vi "Real time state machine - Saccade suppression LED by time2.vi"() -> ()   [LabVIEW 2013]
uses:
  <vilib>/Platform/TimedLoop/XDataNode/timing_clust.ctl
  <vilib>/Platform/TimedLoop/XDataNode/nitl_modes.ctl
  <vilib>/Platform/TimedLoop/XDataNode/wakeup.ctl
  <vilib>/DAQmx/write.llb/DAQmx Write (Digital 1D Bool NChan 1Samp 1Line).vi
  <vilib>/DAQmx/read.llb/DAQmx Read (Analog 1D DBL NChan 1Samp).vi
  <vilib>/DAQmx/write.llb/DAQmx Write (Analog DBL 1Chan 1Samp).vi
  <vilib>/platform/TimedLoop/XDataNode/XDataNode.xnode
  <vilib>/Platform/TimedLoop/XDataNode/XDNodeRunTimeDep.lvlib
panel:
  in  "Local port":u16=9091
  in  "Local IP_This computer":string="192.168.137.2"
  out "ABORT":bool
  out "Initial data received":bool
  out "Busy":bool
  out "Trial Done":bool=TRUE
  in  "Remote port":u16=9090
  in  "Remote IP_Main":string="192.168.137.10"
  out "Trial #":i32=5
  out "Start one trial":bool
  out "RT FIFO (Log)":u32(slide) scale=0.0..50.0
  out "error out":errorcluster
  out "Actual cycle period (uS)":i64=104
  out "# of rewards":i32
  in  "Automatic reward":bool=TRUE
  out "Digital Waveform Graph":digitalwaveform(graph)={"t0"=timestamp(3672173571.3850894 s since 1904-01-01), "dt"=0.0004, "Y"={"transitions"=[], "data"=array25000x3[75000 elements]}, "error"={"status"=FALSE, "code"=37421928, "source"=""}}
  out "shaft encoder":waveform(sgl)(graph)={"t0"=timestamp(3672173571.3850894 s since 1904-01-01), "dt"=0.02, "Y"=array[500 elements]}
  out "Min":dbl=20.0
  out "Sec":dbl=23.69873046875
  out "Trial # (State machine)":u32=6
  out "Current state":T1(ring)
  out "RT FIFO (DISP)":u32(slide) scale=0.0..50.0
  in  "State machine cycle (uS)":i64=200
  in  "Save file to":string="C:\\ni-rt\\LabVIEW Data\\"
  in  "Display length (S)":sgl=10.0
  in  "RT FIFO size":u32=50
  in  "VS filter period (uS)":i32=500
  out "LED?":bool
  out "Pulse amp 0":sgl
  out "Pulse amp 1":sgl
  out "Pulse delay":sgl
  out "Pulse width":sgl
  out "Pulse period (ms)":sgl
  out "Pulse #":sgl
  out "Reward period (uS)":u32
  out "Reward start delay (uS)":u32
  out "Water duration (uS)":u32=30000
  out "Water refractory period (uS)":u32=500000
  out "Shock duration (uS)":u32=10000
  out "Shock refractory period (uS)":u32=1000000
  out "Trial timeout (uS)":u32=3000000
  out "Lick threshold (V)":fxp<+,32,16>=1.600006103515625
  out "Track eye":bool=TRUE
  out "Allow shock":bool
  out "Allow timeout":bool
  out "Manually give water":bool
  out "Manually give shock":bool
  out "VS threshold (V)":fxp<+,32,16>=2.0
  out "VS type":string="test"
  out "File name":string="Test"
  out "Behavior type":string="test"
  out "Save data":bool
  out "Lick reward":bool
  in  "Stop state":bool
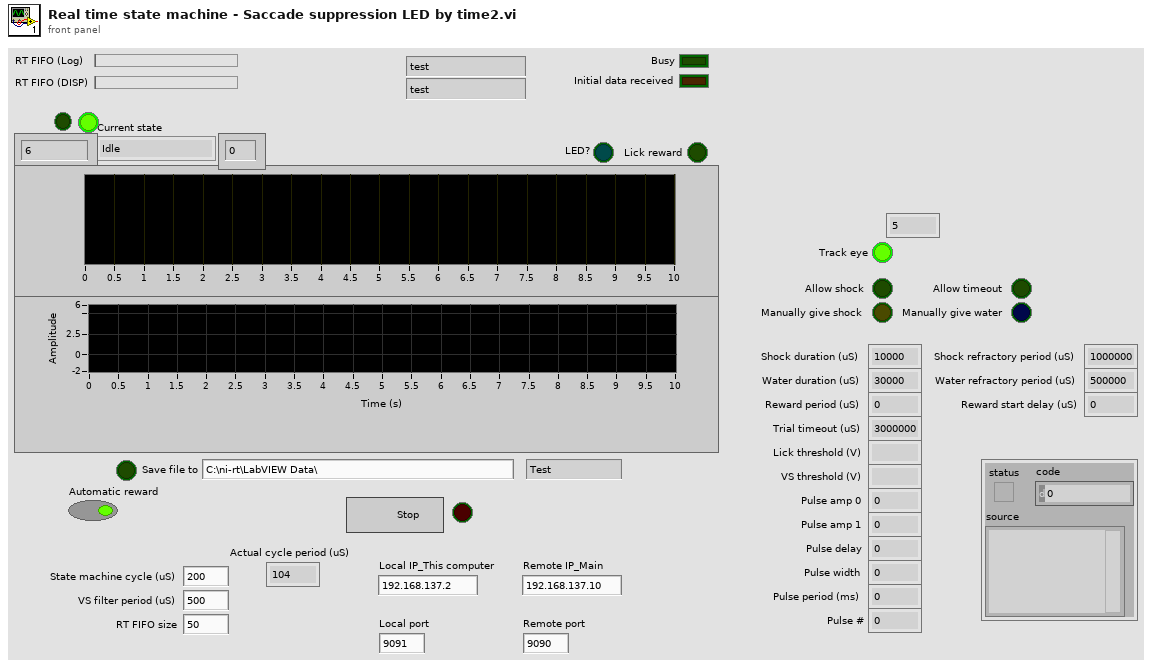
[diagram p1: front panel]
types:
  T1 = enum16{"Idle", "Before VS", "VS", "VS2", "After VS", "Wait for lever press", "Cycle End", "Reward", "Reward Refractory", "Punish", "Punish Refractory", "Exit", "Timeout", "Lick reward"}
  T2 = enum16{"open", "replace", "create", "open or create", "replace or create", "replace or create with confirmation"}
  T3 = typedef "XDNodeRunTimeDep.lvlib/timing_clust.ctl" = cluster{"Expected End [f-1]":u64, "Actual End [f-1]":u64, "Finished Late? [f-1]":bool, "Expected End [i-1]":u64, "Actual End [i-1]":u64, "Finished Late? [i-1]":bool, "Expected Start [i]":u64, "Actual Start [i]":u64, "Expected Start [f]":u64, "Actual Start [f]":u64, "Source Name":string, "Structure Name":string, "Period":i64, "Deadline":i64, "Offset":i64, "Start":i64, "Priority":i32, "Timeout":i32, "Mode":T4, "Wakeup Reason":T5, "Error":errorcluster, "Source Type":string, "Secondary Source Type":string, "Global End Time":u64, "Global Start Time":u64, "Frame Duration":u64, "Iteration Duration":u64, "Assigned CPU":i32, "I/O Scan Engine Mode":u32}
  T4 = typedef "XDNodeRunTimeDep.lvlib/nitl_modes.ctl" = enum32{"No Change", "Process missed periods, maintain original phase", "Discard missed periods, maintain original phase", "Process missed periods, ignore original phase", "Discard missed periods, ignore original phase"}
  T5 = typedef "XDNodeRunTimeDep.lvlib/wakeup.ctl" = enum32{"Normal", "Aborted", "Asynchronous wakeup", "Timing source error", "Timed loop error", "Timeout"}
  T6 = enum16{"big-endian, network order", "native, host order", "little-endian"}
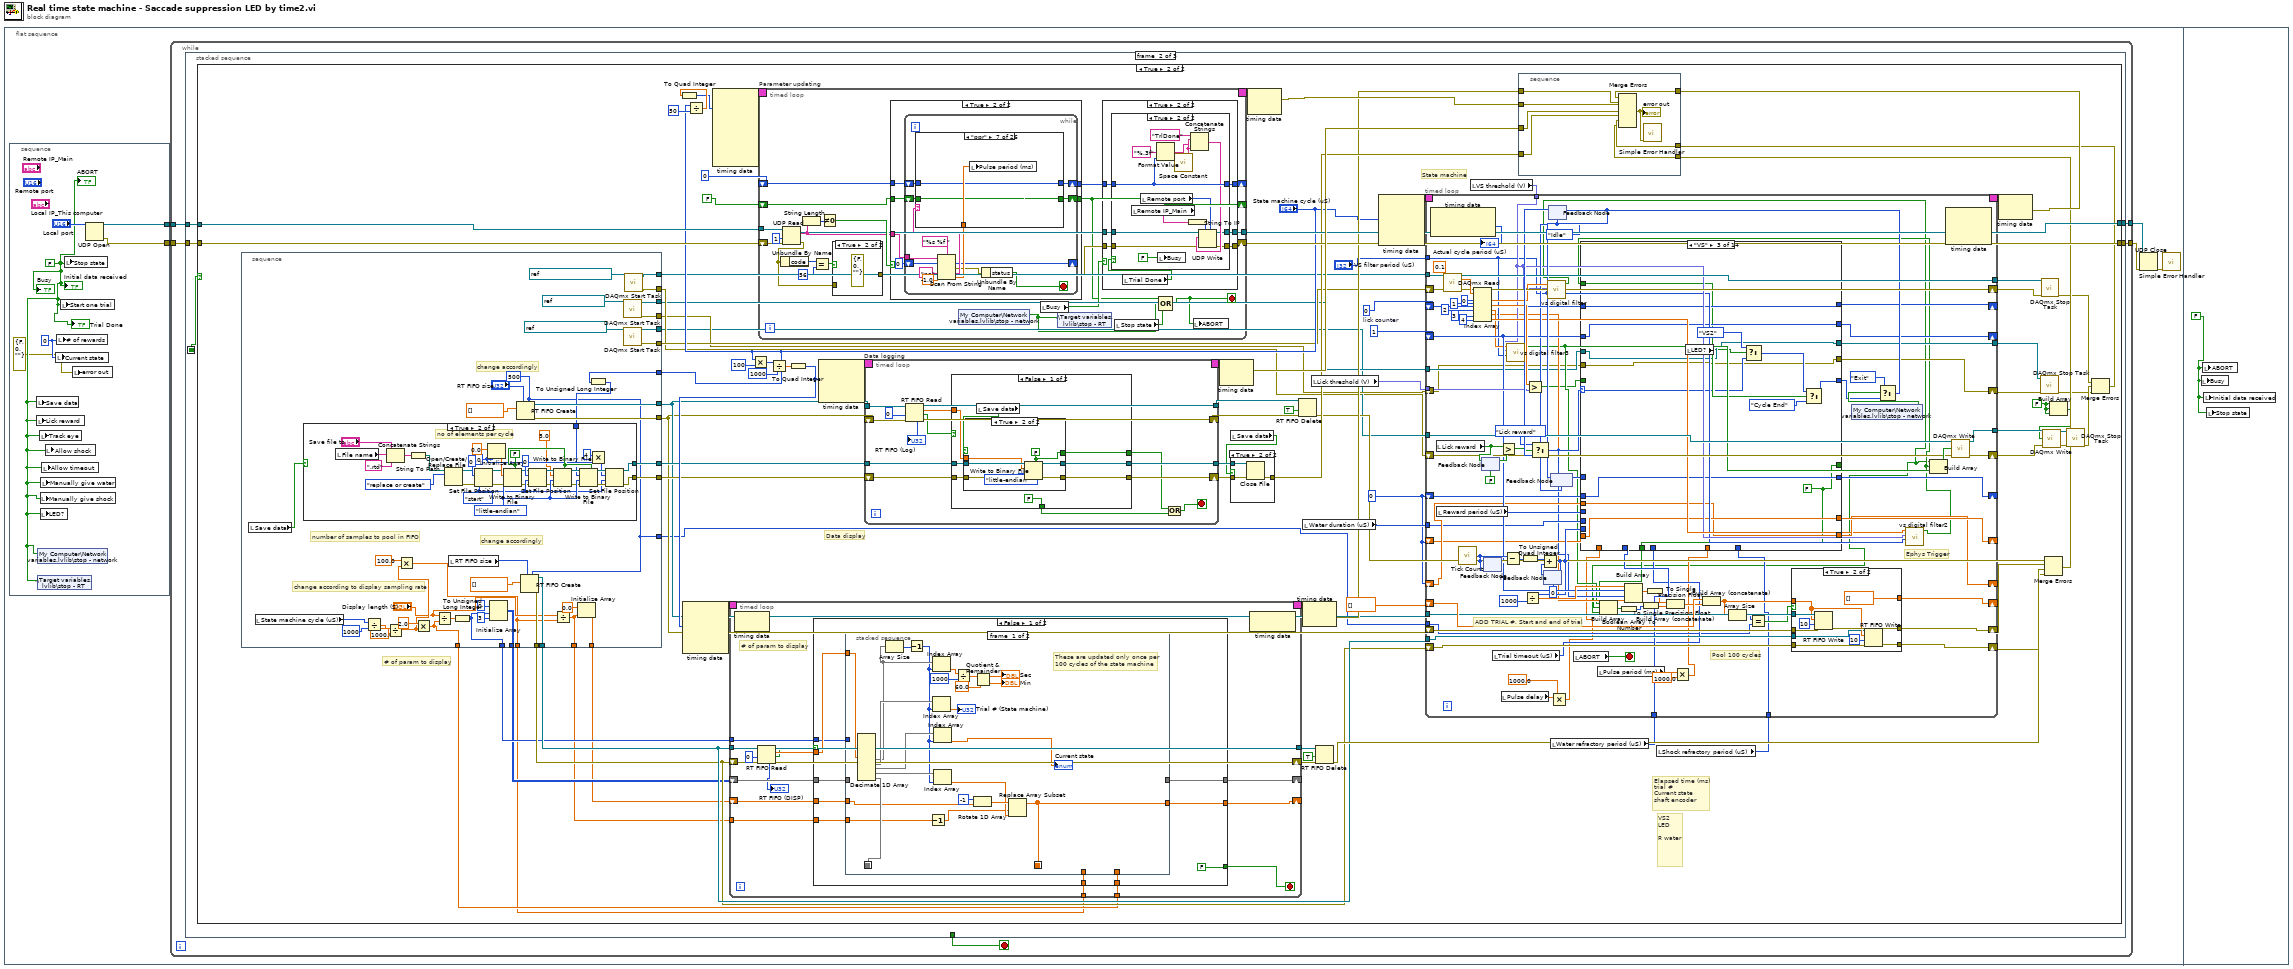
[diagram p0: block diagram]
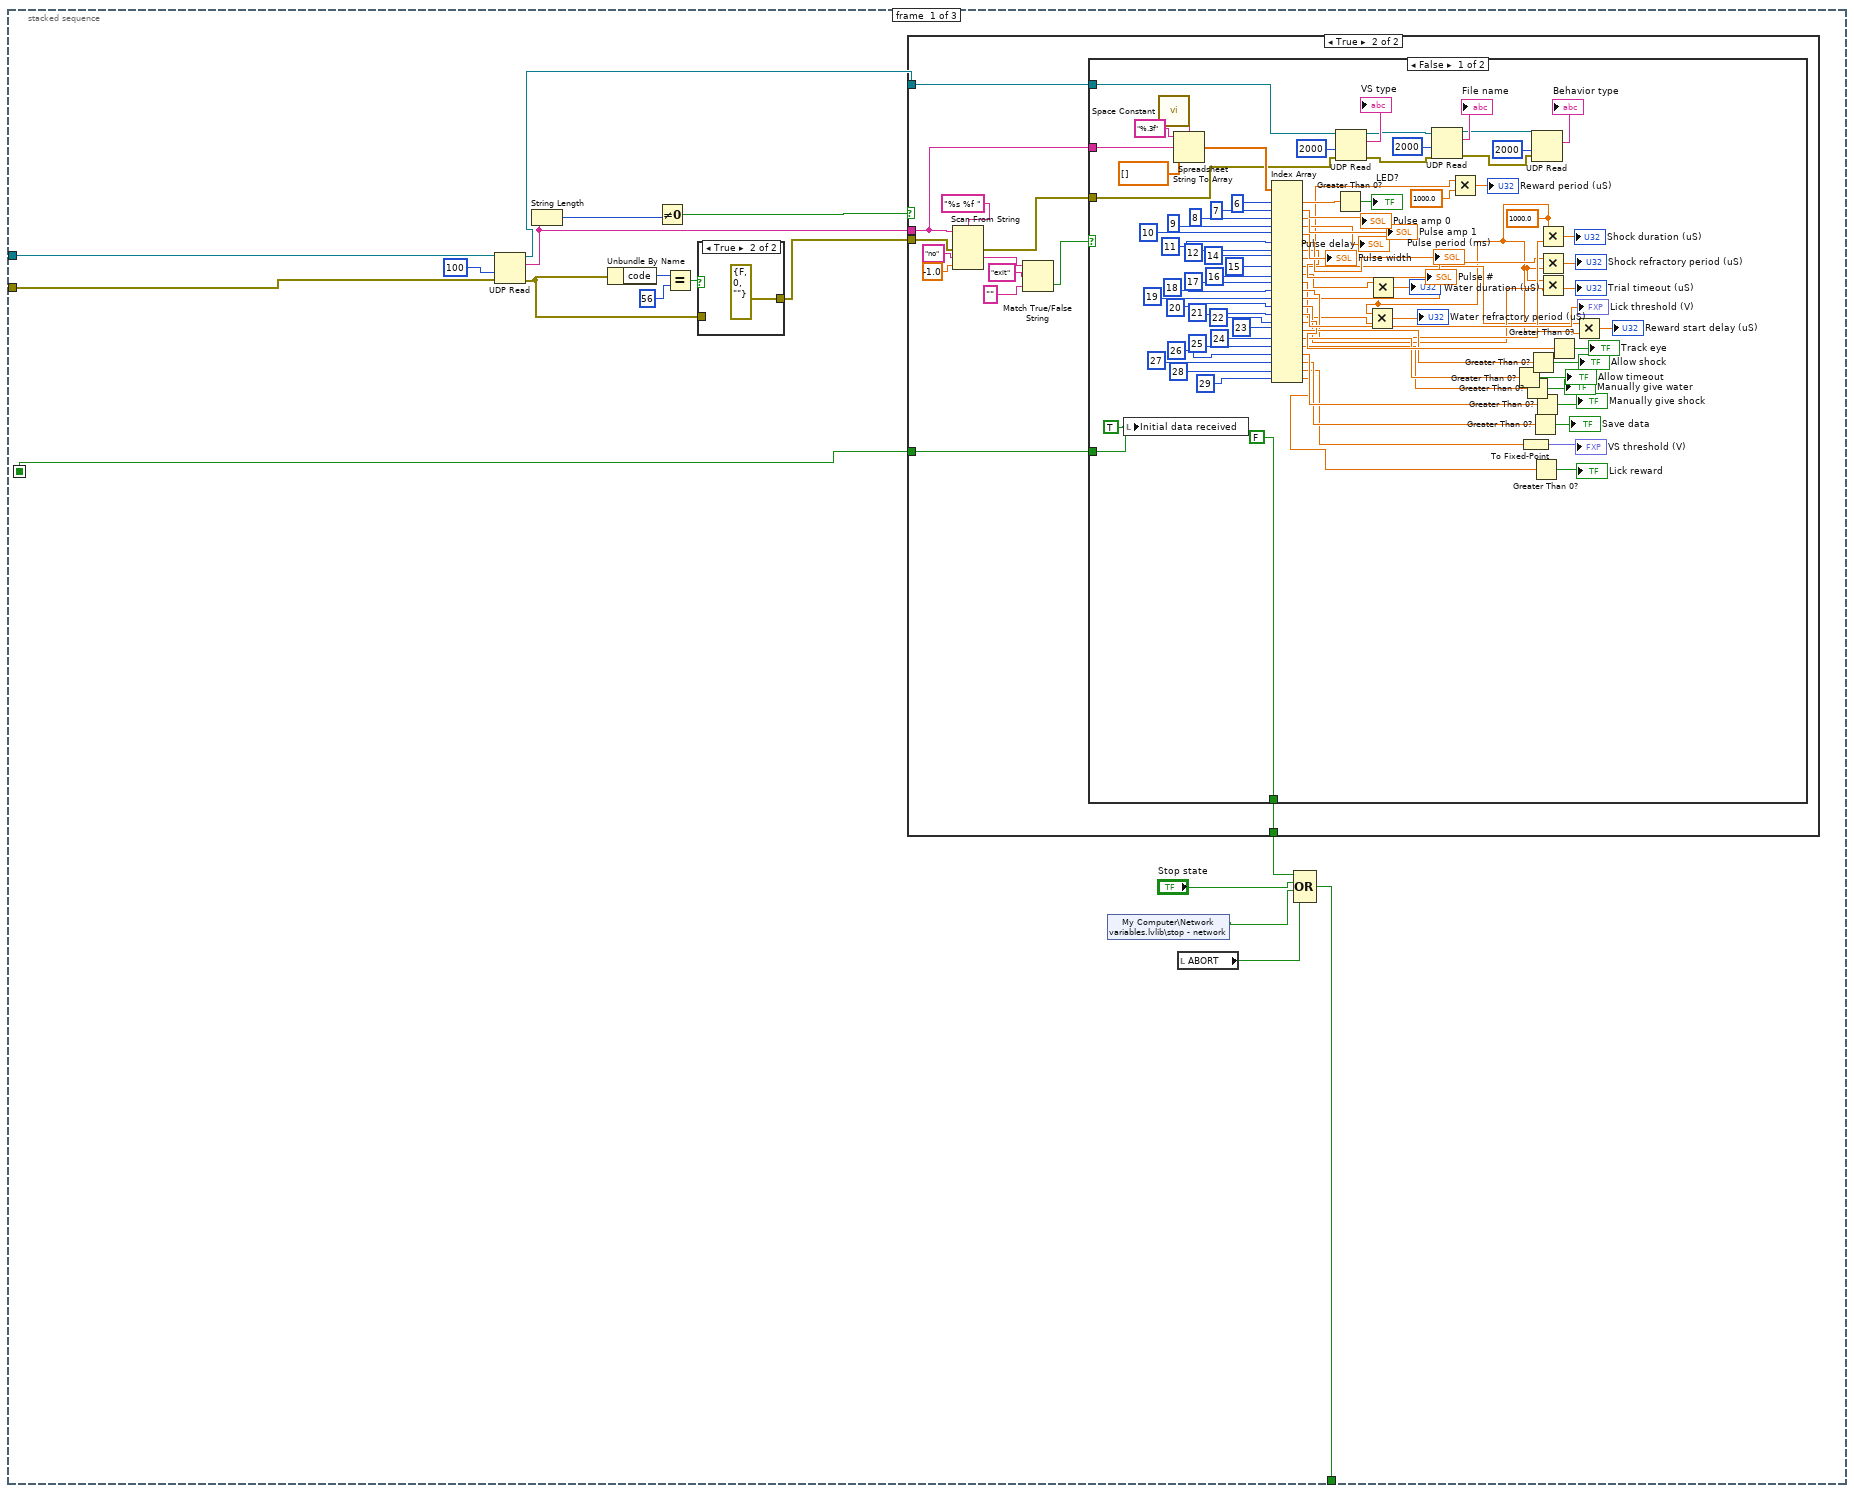
[diagram p2: hidden frame]
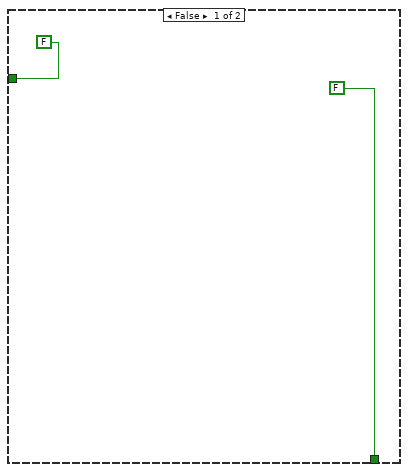
[diagram p3: hidden frame]
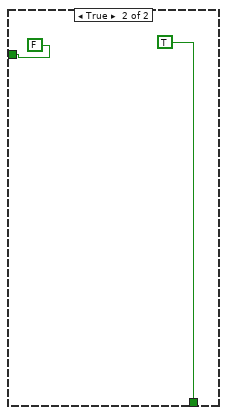
[diagram p4: hidden frame]
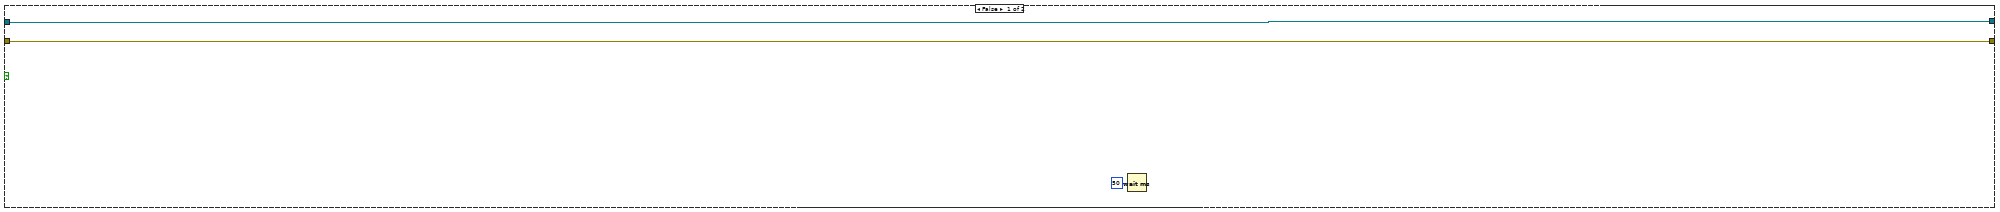
[diagram p6: hidden frame]
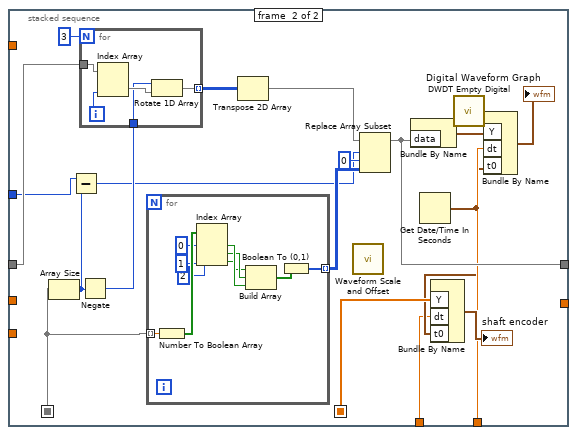
[diagram p9: hidden frame]
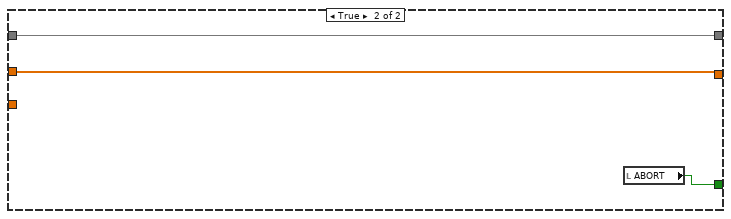
[diagram p10: hidden frame]
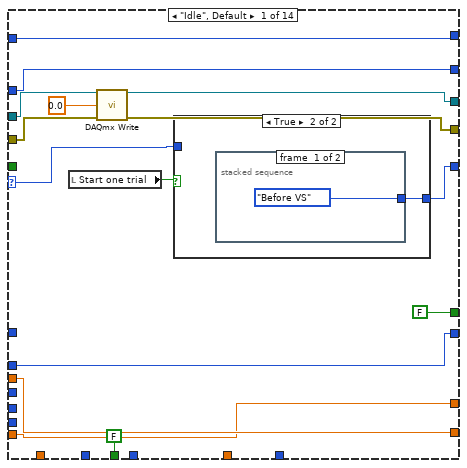
[diagram p11: hidden frame]
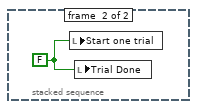
[diagram p13: hidden frame]
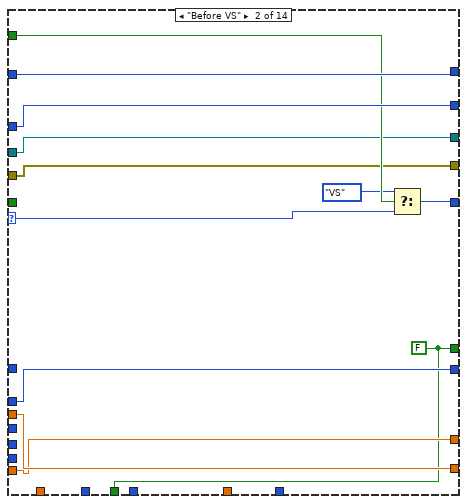
[diagram p14: hidden frame]
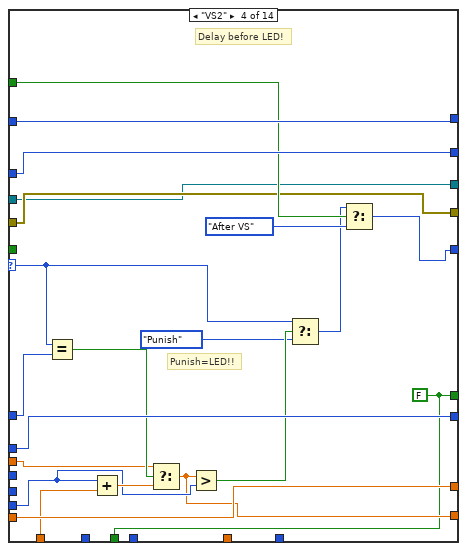
[diagram p15: hidden frame]
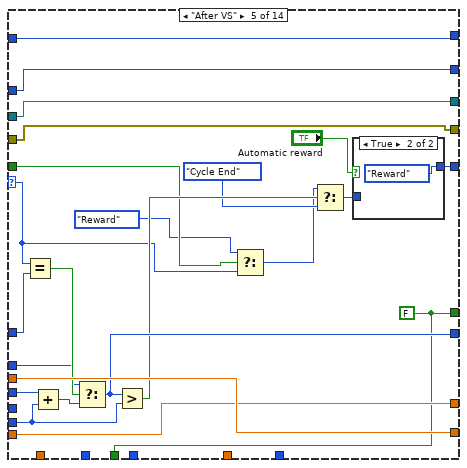
[diagram p16: hidden frame]
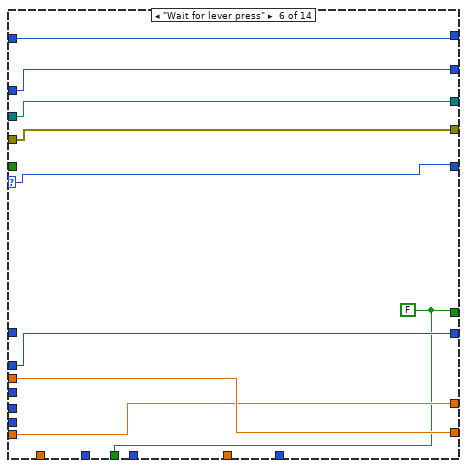
[diagram p18: hidden frame]
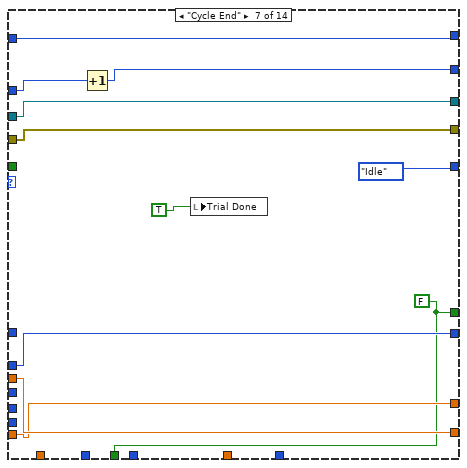
[diagram p19: hidden frame]
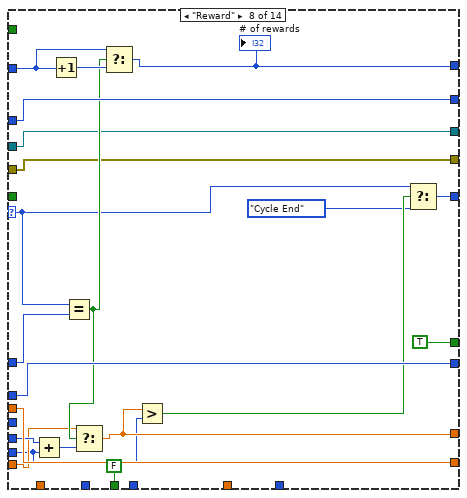
[diagram p20: hidden frame]
diagram:
  n1 = flat-sequence {
    frame #0 {
      n2 = stacked-sequence {
        tunnel: [w995] -> w5
        tunnel: [w994] -> w4
        frame #0 {
          w993 = 0
          w992 = FALSE
          n3 = local write "Save data"(w992) -> ()
          n4 = local write "Lick reward"(w992) -> ()
          n5 = shared-variable "My Computer\\Network variables.lvlib\\stop - network"(w992) -> ()  [unwired: 1 in, 1 out]
          n6 = shared-variable ".\\Target variables.lvlib\\stop - RT"(w992) -> ()  [unwired: 1 in, 1 out]
          n7 = local write "Track eye"(w992) -> ()
          n8 = local write "Manually give shock"(w992) -> ()
          n9 = local write "LED?"(w992) -> ()
          n10 = local write "Manually give water"(w992) -> ()
          n11 = local write "Allow timeout"(w992) -> ()
          n12 = local write "Allow shock"(w992) -> ()
          n13 = local write "Current state"(w993) -> ()
          n14 = local write "# of rewards"(w993) -> ()
          n15 = local write "Start one trial"(w992) -> ()
          n16 = local write "Stop state"(w992) -> ()
          n17 = local write "error out"(errorcluster {"status"=FALSE, "code"=0, "source"=""} ("error out")) -> ()
          n18 = UDP Open(11:"Local port") -> (port=w995:refnum<k16>, 0:w994:errorcluster)  [unwired: 4 in, 1 out]
          "ABORT" <- w992
          "Initial data received" <- w992
          "Busy" <- w992
          "Trial Done" <- w992
        }
      }
      n19 = while {
        tunnel: w5 -> [w10]
        tunnel: w4 -> [w9]
        tunnel: [w8] -> w3
        tunnel: [w7] -> w2
        stop <- w6 stop-if-true
        n20 = stacked-sequence {
          seq-local: [w16 _ _] -> [_ w135 _]
          tunnel: w10 -> [w27 w132 _]
          tunnel: w9 -> [w26 w133 _]
          tunnel: [w15 _ _] -> w6
          tunnel: [_ w134 _] -> w8
          tunnel: [_ w131 _] -> w7
          frame #0 {
            n21 = UDP Read(connection ID=w27, timeout ms (25000)=100, 8:w26) -> (data out=w18:string, error out=w22:errorcluster, 3:w17:refnum<k16>)  [unwired: 1 in, 2 out]
            n22 = String Length(string=w18) -> (length=w21:i32)
            n23 = Unbundle By Name(w22) -> ("code"=w25:i32)
            n24 = Not Equal To 0?(x=w21) -> (x != 0?=w20:bool)
            n25 = Equal?(x=w25, y=56) -> (x = y?=w23:bool)
            n26 = case shown="True" w23 {
              tunnel: w22 -> [w129 _]
              tunnel: [w129 errorcluster {"status"=FALSE, "code"=0, "source"=""} ("error out")] -> w19
              frame False {
              }
              frame True {
              }
            }
            n27 = case shown="True" w20 {
              tunnel: w19 -> [_ w41]
              tunnel: w18 -> [_ w35]
              tunnel: w17 -> [_ w33]
              tunnel: [FALSE w32] -> w14
              tunnel: [FALSE w31] -> w16
              frame False {
              }
              frame True {
                n28 = Scan From String(format string="%s %f ", input string=w35, error in=w41, default 1="no" ("default value 1"), default 2=sgl -1.0 ("default value 1")) -> (error out=w34:errorcluster, output 1=w39:string)  [unwired: 2 in, 2 out]
                n29 = Match True/False String(2:"" ("false string"), 3:"exit" ("true string"), 4:w39) -> (0:w36:bool)  [unwired: 1 out]
                n30 = case shown="False" w36 {
                  tunnel: w35 -> [w123 _]
                  tunnel: w34 -> [w81 _]
                  tunnel: w33 -> [w80 _]
                  tunnel: [FALSE TRUE] -> w32
                  tunnel: [w68 FALSE] -> w31
                  frame False {
                    w49 = sgl 1000.0
                    w68 = TRUE
                    n31 = local write "Initial data received"(w68) -> ()
                    n32 = call <vilib>:"Space Constant.vi"() -> ("String"=w125:string)
                    n33 = Spreadsheet String To Array(delimiter (Tab)=w125, format string="%.3f", spreadsheet string=w123, array type (2D Dbl)=sgl[] []) -> (array=w122:sgl[])
                    n34 = Index Array(array=w122, index #1=6 ("index"), index #2=7 ("index"), index #3=8 ("index"), index #4=9 ("index"), index #5=10 ("index"), index #6=11 ("index"), index #7=12 ("index"), index #8=14 ("index"), index #9=15 ("index"), index #10=16 ("index"), index #11=17 ("index"), index #12=18 ("index"), index #13=19 ("index"), index #14=20 ("index"), index #15=21 ("index"), index #16=22 ("index"), index #17=23 ("index"), index #18=24 ("index"), index #19=25 ("index"), index #20=26 ("index"), index #21=27 ("index"), index #22=28 ("index"), index #23=29 ("index")) -> (element #1=w120:sgl, element #2=→"Pulse amp 0":sgl, element #3=→"Pulse amp 1":sgl, element #4=→"Pulse delay":sgl, element #5=→"Pulse width":sgl, element #6=→"Pulse period (ms)":sgl, element #7=→"Pulse #":sgl, element #8=w64:sgl, element #9=w55:sgl, element #10=w53:sgl, element #11=w51:sgl, element #12=w61:sgl, element #13=w60:sgl, element #14=w57:sgl, element #15=→"Lick threshold (V)":sgl, element #16=w94:sgl, element #17=w91:sgl, element #18=w89:sgl, element #19=w86:sgl, element #20=w84:sgl, element #21=w46:sgl, element #22=w45:sgl, element #23=w44:sgl)
                    n35 = Greater Than 0?(x=w120) -> (x > 0?=→"LED?":bool)
                    n36 = UDP Read(connection ID=w80, timeout ms (25000)=2000, 8:w81) -> (data out=→"VS type":string, error out=w76:errorcluster, 3:w74:refnum<k16>)  [unwired: 1 in, 2 out]
                    n37 = Multiply(x=w49, y=w51) -> (x*y=→"Water refractory period (uS)":sgl)
                    n38 = Multiply(x=w53, y=w49) -> (x*y=→"Water duration (uS)":sgl)
                    n39 = UDP Read(connection ID=w74, timeout ms (25000)=2000, 8:w76) -> (data out=→"File name":string, error out=w72:errorcluster, 3:w71:refnum<k16>)  [unwired: 1 in, 2 out]
                    n40 = Multiply(x=w64, y=sgl 1000.0) -> (x*y=→"Reward period (uS)":sgl)
                    n41 = Greater Than 0?(x=w89) -> (x > 0?=→"Allow timeout":bool)
                    n42 = To Fixed-Point(number=w45) -> (fixed-point=→"VS threshold (V)":fxp<+/-,32,16>)  [unwired: 1 in]
                    n43 = Greater Than 0?(x=w86) -> (x > 0?=→"Manually give water":bool)
                    n44 = Greater Than 0?(x=w91) -> (x > 0?=→"Allow shock":bool)
                    n45 = Greater Than 0?(x=w46) -> (x > 0?=→"Save data":bool)
                    n46 = Greater Than 0?(x=w44) -> (x > 0?=→"Lick reward":bool)
                    n47 = UDP Read(connection ID=w71, timeout ms (25000)=2000, 8:w72) -> (data out=→"Behavior type":string)  [unwired: 1 in, 4 out]
                    n48 = Greater Than 0?(x=w84) -> (x > 0?=→"Manually give shock":bool)
                    n49 = Multiply(x=w49, y=w61) -> (x*y=→"Shock duration (uS)":sgl)
                    n50 = Multiply(x=w60, y=w49) -> (x*y=→"Shock refractory period (uS)":sgl)
                    n51 = Multiply(x=w49, y=w57) -> (x*y=→"Trial timeout (uS)":sgl)
                    n52 = Greater Than 0?(x=w94) -> (x > 0?=→"Track eye":bool)
                    n53 = Multiply(x=w55, y=w49) -> (x*y=→"Reward start delay (uS)":sgl)
                  }
                  frame True {
                  }
                }
              }
            }
            n54 = shared-variable "My Computer\\Network variables.lvlib\\stop - network"() -> (w11:bool)  [unwired: 1 in, 1 out]
            n55 = local read "ABORT"() -> (w12:bool)
            n56 = Compound Arithmetic op=OR(w14, "Stop state", w11, w12) -> (w15:bool)
          }
          frame #1 {
            n57 = case shown="True" w135 {
              tunnel: w133 -> [w138 w215]
              tunnel: [w138 w207] -> w134
              tunnel: w132 -> [w137 w214]
              tunnel: [w137 w206] -> w131
              frame False {
                n58 = Wait (ms)(milliseconds to wait=u32 50) -> ()  [unwired: 1 out]
              }
              frame True {
                w159 = FALSE
                w195 = 0  # lick counter
                w152 = 0
                # "VS2\nLED\n\nR water"
                # "# of param to display"
                # "Data display"
                # "Elapsed time (ms)\ntrial #\nCurrent state\nshaft encoder"
                # "State machine"
                n59 = stacked-sequence {
                  tunnel: [w267] -> w180
                  tunnel: [w266] -> w179
                  tunnel: [w263] -> w178
                  tunnel: [w262] -> w177
                  tunnel: [w248] -> w160
                  tunnel: [w243] -> w176
                  tunnel: [w254] -> w175
                  tunnel: "State machine cycle (uS)" -> [w247]
                  tunnel: [w251] -> w173
                  tunnel: [w250] -> w172
                  tunnel: [w245] -> w151
                  tunnel: [w242] -> w150
                  tunnel: [w238] -> w149
                  tunnel: [w237] -> w148
                  tunnel: [w235] -> w144
                  tunnel: [w234] -> w143
                  tunnel: [w232] -> w142
                  tunnel: [w231] -> w141
                  tunnel: [w229] -> w140
                  tunnel: [w228] -> w139
                  frame #0 {
                    w245 = u32 500 ("elements in array (1)")
                    # "number of samples to pool in FIFO"
                    # "change according to display sampling rate"
                    # "change accordingly"
                    # "change accordingly"
                    n60 = local read "Save data"() -> (w268:bool)
                    n61 = local read "State machine cycle (uS)"() -> (w255:i64)
                    n62 = Divide(x=w255, y=u32 1000) -> (x/y=w257:dbl)
                    n63 = Divide(x=w257, y=1000.0) -> (x/y=w240:dbl)
                    n64 = Multiply(x=100.0, y=w240) -> (x*y=w238:dbl)
                    n65 = Multiply(x=2.0, y=w240) -> (x*y=w248:dbl)
                    n66 = Divide(x="Display length (S)", y=w248) -> (x/y=w260:dbl)
                    n67 = local read "RT FIFO size"() -> (w265:u32)
                    n68 = To Unsigned Long Integer(number=w260) -> (unsigned 32bit integer=w243:u32)
                    n69 = Initialize Array(u8 0 ("element"), w243, 3 ("dimension size")) -> (w254:u8[][])
                    n70 = RT FIFO Create(1:sgl[] [], 4:"RT FIFO size", 6:w245) -> (8:w251:refnum<k33>, 11:w250:errorcluster)  [unwired: 5 in, 1 out]
                    n71 = RT FIFO Create(1:sgl[] [], 4:w265, 6:w245) -> (8:w263:refnum<k33>, 11:w262:errorcluster)  [unwired: 5 in, 1 out]
                    n72 = Divide(x="Display length (S)", y=w238) -> (x/y=w237:dbl)
                    n73 = Initialize Array(sgl 0.0 ("element"), w237) -> (w242:sgl[])
                    n74 = To Unsigned Long Integer(number=w247) -> (unsigned 32bit integer=w246:u32)
                    n75 = case shown="True" w268 {
                      tunnel: [_ w272] -> w267
                      tunnel: [_ w271] -> w266
                      tunnel: w246 -> [_ w270]
                      frame False {
                      }
                      frame True {
                        w293 = FALSE
                        w286 = 10 ("dimension size")
                        w294 = T6."little-endian" ("byte order (0:big-endian, network order)")
                        w285 = enum16{"start", "end", "current"}."start" ("from (0:start)")
                        # "no of elements per cycle"
                        n76 = local read "File name"() -> (w296:string)
                        n77 = Concatenate Strings("Save file to", w296, ".rtd" ("string")) -> (w299:string)
                        n78 = String To Path(string=w299) -> (path=w300:path)
                        n79 = Open/Create/Replace File(file path (use dialog)=w300, operation (0:open)=T2."replace or create") -> (refnum out=w273:refnum<file>, error out=w274:errorcluster)  [unwired: 4 in, 1 out]
                        n80 = Set File Position(offset (in bytes) (0)=i64 0, refnum=w273, from (0:start)=w285, error in=w274) -> (refnum out=w276:refnum<file>, error out=w277:errorcluster)
                        n81 = Initialize Array(sgl 0.0 ("element"), w286) -> (w279:sgl[])
                        n82 = Write to Binary File(file (use dialog)=w276, data=w279, error in=w277, 5:w293, 9:w294) -> (refnum out=w281:refnum<file>, error out=w280:errorcluster)  [unwired: 1 in, 1 out]
                        n83 = Set File Position(offset (in bytes) (0)=i64 0, refnum=w281, from (0:start)=w285, error in=w280) -> (refnum out=w283:refnum<file>, error out=w284:errorcluster)
                        n84 = Write to Binary File(file (use dialog)=w283, data=sgl 5.0, error in=w284, 5:w293, 9:w294) -> (refnum out=w291:refnum<file>, error out=w289:errorcluster)  [unwired: 1 in, 1 out]
                        n85 = Write to Binary File(file (use dialog)=w291, data=w270, error in=w289, 5:w293, 9:w294) -> (refnum out=w292:refnum<file>, error out=w290:errorcluster)  [unwired: 1 in, 1 out]
                        n86 = Multiply(x=4, y=w286) -> (x*y=w288:i32)
                        n87 = Set File Position(offset (in bytes) (0)=w288, refnum=w292, from (0:start)=w285, error in=w290) -> (refnum out=w271:refnum<file>, error out=w272:errorcluster)
                      }
                    }
                    n88 = call <vilib>:"DAQmx Start Task.vi"("task/channels in"=refnum<k21> "LED analog out" ("DAQmx Task Name")) -> ("task out"=w232:refnum<k21>, "error out"=w231:errorcluster)  [unwired: 13 in]
                    n89 = call <vilib>:"DAQmx Start Task.vi"("task/channels in"=refnum<k21> "Digital_write_saccade" ("DAQmx Task Name")) -> ("task out"=w229:refnum<k21>, "error out"=w228:errorcluster)  [unwired: 13 in]
                    n90 = call <vilib>:"DAQmx Start Task.vi"("task/channels in"=refnum<k21> "Analog_read_saccade" ("DAQmx Task Name")) -> ("task out"=w235:refnum<k21>, "error out"=w234:errorcluster)  [unwired: 13 in]
                  }
                }
                n91 = Divide(x="State machine cycle (uS)", y=i64 50) -> (x/y=w185:dbl)
                n92 = To Quad Integer(1:w185) -> (0:w184:i64)
                n93 = node-c288 ("Input Node")(w184) -> (w223:T3)  [unwired: 6 in]
                n94 = Multiply(x="State machine cycle (uS)", y=u32 100) -> (x*y=w188:i64)
                n95 = timed-loop "Parameter updating" {
                  timing: w223 -> [_]
                  timing-out: [_] -> w222
                  tunnel: w214 -> [w828]
                  shift-right: [w813] -> w207
                  shift-left: w215 -> [w829]
                  shift-right: [w816] -> _
                  shift-left: 0 -> [w819]
                  tunnel: [w812] -> w206
                  shift-right: [w810] -> _
                  shift-left: FALSE -> [w820]
                  stop <- w811 stop-if-true
                  n96 = UDP Read(connection ID=w828, timeout ms (25000)=1, 8:w829) -> (data out=w821:string, error out=w824:errorcluster, 3:w814:refnum<k16>)  [unwired: 1 in, 2 out]
                  n97 = Unbundle By Name(w824) -> ("code"=w827:i32)
                  n98 = String Length(string=w821) -> (length=w823:i32)
                  n99 = Equal?(x=w827, y=56) -> (x = y?=w825:bool)
                  n100 = Not Equal To 0?(x=w823) -> (x != 0?=w822:bool)
                  n101 = case shown="True" w825 {
                    tunnel: w824 -> [w981 _]
                    tunnel: [w981 errorcluster {"status"=FALSE, "code"=0, "source"=""} ("error out")] -> w815
                    frame False {
                    }
                    frame True {
                    }
                  }
                  n102 = case shown="True" w822 {
                    tunnel: w821 -> [_ w864]
                    tunnel: w820 -> [w857 w863]
                    tunnel: w819 -> [w858 w862]
                    tunnel: [w858 w861] -> w817
                    tunnel: [w857 w860] -> w810
                    frame False {
                    }
                    frame True {
                      n103 = while {
                        tunnel: w864 -> [w876]
                        shift-right: [w872] -> w860
                        shift-left: w863 -> [w873]
                        shift-right: [w871] -> w861
                        shift-left: w862 -> [w870]
                        shift-right: [w866] -> _
                        shift-left: u32 0 -> [w867]
                        stop <- w868 stop-if-true
                        n104 = Scan From String(format string="%s %f ", input string=w876, initial scan location=w867, default 1="no" ("default value 1"), default 2=-1.0 ("default value 2")) -> (offset past scan=w866:u32, error out=w869:errorcluster, output 1=w875:string, output 2=w874:dbl)  [unwired: 1 in, 1 out]
                        n105 = case shown="\"ppr\"" w875 {
                          tunnel: w874 -> [_ w883 w887 w890 w893 w896 w899 w902 w904 w908 w913 w919 w924 w929 w934 w940 w943 w947 w952 w955 w959 w963 w966 w970 _ _]
                          tunnel: w873 -> [w880 w881 w885 w888 w891 w894 w897 w900 w906 w911 w916 w921 w926 w931 w936 w938 w941 w945 w949 w953 w957 w961 w967 w971 w974 w979]
                          tunnel: [w880 w881 w885 w888 w891 w894 w897 w900 w906 w911 w916 w921 w926 w931 w936 w938 w941 w945 w949 w953 w957 w961 w967 w971 w974 w978] -> w872
                          tunnel: [w879 w882 w886 w889 w892 w895 w898 w901 w907 w912 w917 w922 w927 w932 w937 w939 w942 w946 w950 w954 w958 w962 w968 w972 w975 w977] -> w871
                          tunnel: w870 -> [w879 w882 w886 w889 w892 w895 w898 w901 w907 w912 w917 w922 w927 w932 w937 w939 w942 w946 w950 w954 w958 w962 w968 w972 w976 w977]
                          frame "no", Default {
                          }
                          frame "led" {
                            n106 = Greater Than 0?(x=w883) -> (x > 0?=w884:bool)
                            n107 = local write "LED?"(w884) -> ()
                          }
                          frame "pai" {
                            n108 = local write "Pulse amp 0"(w887) -> ()
                          }
                          frame "paf" {
                            n109 = local write "Pulse amp 1"(w890) -> ()
                          }
                          frame "pdl" {
                            n110 = local write "Pulse delay"(w893) -> ()
                          }
                          frame "pwd" {
                            n111 = local write "Pulse width"(w896) -> ()
                          }
                          frame "ppr" {
                            n112 = local write "Pulse period (ms)"(w899) -> ()
                          }
                          frame "pnm" {
                            n113 = local write "Pulse #"(w902) -> ()
                          }
                          frame "rwp" {
                            n114 = Multiply(x=1000.0, y=w904) -> (x*y=w903:dbl)
                            n115 = local write "Reward period (uS)"(w903) -> ()
                          }
                          frame "rwd" {
                            n116 = Multiply(x=1000.0, y=w908) -> (x*y=w909:dbl)
                            n117 = local write "Reward start delay (uS)"(w909) -> ()
                          }
                          frame "wdr" {
                            n118 = Multiply(x=1000.0, y=w913) -> (x*y=w914:dbl)
                            n119 = local write "Water duration (uS)"(w914) -> ()
                          }
                          frame "wre" {
                            n120 = Multiply(x=1000.0, y=w919) -> (x*y=w918:dbl)
                            n121 = local write "Water refractory period (uS)"(w918) -> ()
                          }
                          frame "shd" {
                            n122 = Multiply(x=1000.0, y=w924) -> (x*y=w923:dbl)
                            n123 = local write "Shock duration (uS)"(w923) -> ()
                          }
                          frame "shr" {
                            n124 = Multiply(x=1000.0, y=w929) -> (x*y=w928:dbl)
                            n125 = local write "Shock refractory period (uS)"(w928) -> ()
                          }
                          frame "tto" {
                            n126 = Multiply(x=1000.0, y=w934) -> (x*y=w933:dbl)
                            n127 = local write "Trial timeout (uS)"(w933) -> ()
                          }
                          frame "lkt" {
                            n128 = local write "Lick threshold (V)"(w940) -> ()
                          }
                          frame "etk" {
                            n129 = Greater Than 0?(x=w943) -> (x > 0?=w944:bool)
                            n130 = local write "Track eye"(w944) -> ()
                          }
                          frame "ash" {
                            n131 = Greater Than 0?(x=w947) -> (x > 0?=w948:bool)
                            n132 = local write "Allow shock"(w948) -> ()
                          }
                          frame "ato" {
                            n133 = Greater Than 0?(x=w952) -> (x > 0?=w951:bool)
                            n134 = local write "Allow timeout"(w951) -> ()
                          }
                          frame "gwt" {
                            n135 = Greater Than 0?(x=w955) -> (x > 0?=w956:bool)
                            n136 = local write "Manually give water"(w956) -> ()
                          }
                          frame "gsh" {
                            n137 = Greater Than 0?(x=w959) -> (x > 0?=w960:bool)
                            n138 = local write "Manually give shock"(w960) -> ()
                          }
                          frame "sav" {
                            n139 = Greater Than 0?(x=w963) -> (x > 0?=w964:bool)
                            n140 = local write "Save data"(w964) -> ()
                          }
                          frame "vsh" {
                            n141 = To Fixed-Point(number=w966) -> (fixed-point=w965:fxp<+/-,32,16>)  [unwired: 1 in]
                            n142 = local write "VS threshold (V)"(w965) -> ()
                          }
                          frame "rew" {
                            n143 = Greater Than 0?(x=w970) -> (x > 0?=w969:bool)
                            n144 = local write "Lick reward"(w969) -> ()
                          }
                          frame "start" {
                            w973 = TRUE
                            n145 = Increment(x=w976) -> (x+1=w975:i32)
                            "Trial #" <- w975
                            n146 = local write "Busy"(w973) -> ()
                            "Start one trial" <- w973
                          }
                          frame "stop" {
                            n147 = Or(x=w979, y=TRUE) -> (x .or. y?=w978:bool)
                          }
                        }
                        n148 = Unbundle By Name(w869) -> ("status"=w868:bool)
                      }
                    }
                  }
                  n149 = shared-variable "My Computer\\Network variables.lvlib\\stop - network"() -> (w808:bool)  [unwired: 1 in, 1 out]
                  n150 = local read "Busy"() -> (w818:bool)
                  n151 = shared-variable ".\\Target variables.lvlib\\stop - RT"(w808) -> ()  [unwired: 1 in, 1 out]
                  n152 = case shown="True" w818 {
                    tunnel: w817 -> [w832 w838]
                    tunnel: [w832 w837] -> w816
                    tunnel: w815 -> [w830 w836]
                    tunnel: w814 -> [w831 w835]
                    tunnel: [w830 w834] -> w813
                    tunnel: [w831 w833] -> w812
                    frame False {
                    }
                    frame True {
                      n153 = local read "Trial Done"() -> (w839:bool)
                      n154 = case shown="True" w839 {
                        tunnel: [w842 w850] -> w837
                        tunnel: w838 -> [w842 w850]
                        tunnel: w836 -> [w841 w847]
                        tunnel: w835 -> [w840 w846]
                        tunnel: [w841 w844] -> w834
                        tunnel: [w840 w843] -> w833
                        frame False {
                        }
                        frame True {
                          n155 = local read "Remote IP_Main"() -> (w855:string)
                          n156 = local read "Remote port"() -> (w854:u16)
                          n157 = Format Value(format string="%.3f", value (0)=w850) -> (output string=w849:string)  [unwired: 1 in]
                          n158 = local write "Busy"(FALSE) -> ()
                          n159 = call <vilib>:"Space Constant.vi"() -> ("String"=w852:string)
                          n160 = String To IP(1:w855) -> (0:w856:u32)
                          n161 = Concatenate Strings("TrlDone" ("data in"), w852, w849, w852) -> (w848:string)
                          n162 = UDP Write(address=w856, port or service name=w854, connection ID=w846, data in=w848, 8:w847) -> (error out=w844:errorcluster, 3:w843:refnum<k16>)  [unwired: 1 in]
                        }
                      }
                    }
                  }
                  n163 = local read "Stop state"() -> (w809:bool)
                  n164 = Compound Arithmetic op=OR(w810, w808, w809) -> (w811:bool)
                  n165 = local write "ABORT"(w811) -> ()
                }
                n166 = Divide(x=w188, y=u32 1000) -> (x/y=w183:dbl)
                n167 = To Quad Integer(1:w183) -> (0:w182:i64)
                n168 = node-c288(w182) -> (w209:T3)  [unwired: 3 in]
                n169 = timed-loop {
                  timing: w209 -> [_]
                  timing-out: [_] -> w208
                  shift-right: [w314] -> w193
                  shift-left: w177 -> [w315]
                  tunnel: w178 -> [w317]
                  tunnel: [w316] -> w194
                  tunnel: w176 -> [w309]
                  shift-right: [w308] -> _
                  shift-left: w175 -> [w310]
                  tunnel: w160 -> [w307]
                  shift-right: [w303] -> _
                  shift-left: w150 -> [w304]
                  tunnel: w149 -> [w302]
                  tunnel: w148 -> [w301]
                  stop <- w305 stop-if-true
                  # "# of param to display"
                  n170 = node-c288() -> ()  [unwired: 1 in, 1 out]
                  n171 = RT FIFO Read(0:w317, 2:0 ("timeout in ms (0)"), 3:w315) -> (7:→"RT FIFO (DISP)":u32, 8:w316:refnum<k33>, 9:w312:sgl[], 10:w311:bool, 11:w314:errorcluster)  [unwired: 1 in]
                  n172 = case shown="False" w311 {
                    tunnel: w312 -> [w327 _]
                    tunnel: w310 -> [w326 w388]
                    tunnel: w309 -> [w325 _]
                    tunnel: [w324 w388] -> w308
                    tunnel: w307 -> [w323 _]
                    tunnel: [FALSE w387] -> w305
                    tunnel: w304 -> [w321 w386]
                    tunnel: [w320 w386] -> w303
                    tunnel: w302 -> [w319 _]
                    tunnel: w301 -> [w318 _]
                    frame False {
                      n173 = stacked-sequence {
                        seq-local: [w337 _] -> [_ w367]
                        seq-local: [w329 _] -> [_ w353]
                        tunnel: w327 -> [w350 _]
                        tunnel: w326 -> [_ w369]
                        tunnel: w325 -> [_ w362]
                        tunnel: [_ w359] -> w324
                        tunnel: w323 -> [_ w354]
                        tunnel: w321 -> [w334 _]
                        tunnel: [w329 _] -> w320
                        tunnel: w319 -> [_ w351]
                        tunnel: w318 -> [w328 _]
                        frame #0 {
                          # "These are updated only once per \n100 cycles of the state machine"
                          n174 = Decimate 1D Array(w350) -> (w339:sgl[], w340:sgl[], w341:sgl[], w336:sgl[], w337:sgl[])  [unwired: 5 out]
                          n175 = Array Size(array=w339) -> (size(s)=w349:i32)
                          n176 = Decrement(x=w349) -> (x-1=w335:i32)
                          n177 = Decrement(x=w328) -> (x-1=w330:dbl)
                          n178 = Index Array(array=w339, index=w335) -> (element=w348:sgl)
                          n179 = Index Array(array=w340, index=w335) -> (element=→"Trial # (State machine)":sgl)
                          n180 = Index Array(array=w341, index=w335) -> (element=→"Current state":sgl)
                          n181 = Index Array(array=w336, index=w335) -> (element=w332:sgl)
                          n182 = Divide(x=w348, y=u32 1000) -> (x/y=w346:sgl)
                          n183 = Rotate 1D Array(1:w334, 2:-1 ("n")) -> (0:w333:sgl[])
                          n184 = Quotient & Remainder(x=w346, y=60.0) -> (x-y*floor(x/y)=→"Sec":dbl, floor(x/y)=→"Min":dbl)
                          n185 = Replace Array Subset(array=w333, new element=w332, index=w330) -> (w329:sgl[])
                        }
                        frame #1 {
                          n186 = Array Size(array=w367) -> (size(s)=w361:i32)
                          n187 = Subtract(x=w362, y=w361) -> (x-y=w360:u32)
                          n188 = Negate(x=w361) -> (-x=w368:i32)
                          n189 = for {
                            N: 3 -> [_]
                            tunnel: w369 -> [w385]
                            tunnel: w368 -> [w382]
                            tunnel: [w381] -> w365 mode=indexing
                            i -> [w384]
                            n190 = Index Array(array=w385, index (col)=w384) -> (element=w383:u8[])  [unwired: 1 in]
                            n191 = Rotate 1D Array(1:w383, 2:w382) -> (0:w381:u8[])
                          }
                          n192 = for {
                            tunnel: w367 -> [w380] mode=indexing
                            tunnel: [w374] -> w366 mode=indexing
                            n193 = Number To Boolean Array(number=w380) -> (Boolean array=w379:bool[])
                            n194 = Index Array(array=w379, index #1=0 ("index"), index #2=1 ("index"), index #3=2 ("index")) -> (element #1=w373:bool, element #2=w372:bool, element #3=w371:bool)
                            n195 = Build Array(w371, w372, w373) -> (w375:bool[])
                            n196 = Boolean To (0,1)(Boolean=w375) -> (0, 1=w374:i16[])
                          }
                          n197 = Transpose 2D Array(2D array=w365) -> (transposed array=w364:u8[][])
                          n198 = call <vilib>:"Waveform Scale and Offset.vi"() -> ()  [unwired: 10 in, 2 out]
                          n199 = Replace Array Subset(array=w364, new element=w366, index (row)=w360, index (col)=0 ("disabled index (col)")) -> (w359:u8[][])
                          n200 = Bundle By Name("data"=w359) -> (w358:digitaldata)  [unwired: 1 in]
                          n201 = Get Date/Time In Seconds() -> (seconds since 1Jan1904=w352:timestamp)
                          n202 = Bundle By Name("Y"=w353, "dt"=w351, "t0"=w352) -> (→"shaft encoder":waveform(sgl))  [unwired: 1 in]
                          n203 = call <vilib>:"DWDT Empty Digital.vi"() -> ("digital waveform out"=w357:digitalwaveform)  [unwired: 5 in]
                          n204 = Bundle By Name(cluster=w357, "Y"=w358, "dt"=w354, "t0"=w352) -> (→"Digital Waveform Graph":digitalwaveform)
                        }
                      }
                    }
                    frame True {
                      n205 = local read "ABORT"() -> (w387:bool)
                    }
                  }
                  n206 = node-c288() -> ()  [unwired: 1 in, 1 out]
                }
                n207 = node-c288 ("Input Node")(w182) -> (w221:T3)  [unwired: 2 in]
                n208 = timed-loop "Data logging" {
                  timing: w221 -> [_]
                  timing-out: [_] -> w220
                  tunnel: [w777] -> w216
                  tunnel: w179 -> [w775]
                  tunnel: w173 -> [w772]
                  shift-right: [w771] -> w198
                  shift-left: w172 -> [w773]
                  tunnel: [w769] -> w196
                  shift-right: [w776] -> w217
                  shift-left: w180 -> [w774]
                  stop <- w765 stop-if-true
                  n209 = RT FIFO Read(0:w772, 2:0 ("timeout in ms (0)"), 3:w773) -> (7:→"RT FIFO (Log)":u32, 8:w769:refnum<k33>, 9:w767:sgl[], 10:w768:bool, 11:w771:errorcluster)  [unwired: 1 in]
                  n210 = case shown="False" w768 {
                    tunnel: [w785 w798] -> w777
                    tunnel: [w784 w799] -> w776
                    tunnel: w775 -> [w783 w798]
                    tunnel: w774 -> [w782 w799]
                    tunnel: w767 -> [w780 _]
                    tunnel: [FALSE w796] -> w763
                    tunnel: [w778 FALSE] -> w764
                    frame False {
                      n211 = local read "Save data"() -> (w781:bool)
                      n212 = case shown="True" w781 {
                        tunnel: [w788 w795] -> w785
                        tunnel: [w787 w794] -> w784
                        tunnel: w783 -> [w788 w793]
                        tunnel: w782 -> [w787 w792]
                        tunnel: w780 -> [_ w791]
                        tunnel: [w786 w789] -> w778
                        frame False {
                          n213 = local read "ABORT"() -> (w786:bool)
                        }
                        frame True {
                          w789 = FALSE
                          n214 = Write to Binary File(file (use dialog)=w793, data=w791, error in=w792, 5:w789, 9:T6."little-endian" ("byte order (0:big-endian, network order)")) -> (refnum out=w795:refnum<file>, error out=w794:errorcluster)  [unwired: 1 in, 1 out]
                        }
                      }
                    }
                    frame True {
                      n215 = local read "ABORT"() -> (w796:bool)
                    }
                  }
                  n216 = Or(x=w764, y=w763) -> (x .or. y?=w765:bool)
                }
                n217 = node-c288 ("Output Node")(w220) -> (w219:errorcluster)
                n218 = local read "Save data"() -> (w169:bool)
                n219 = case shown="True" w169 {
                  tunnel: w217 -> [w224 w227]
                  tunnel: w216 -> [_ w226]
                  tunnel: [w224 w225] -> w205
                  frame False {
                  }
                  frame True {
                    n220 = Close File(refnum=w226, error in=w227) -> (error out=w225:errorcluster)  [unwired: 1 out]
                  }
                }
                n221 = node-c288 ("Output Node")(w222) -> (w218:errorcluster)
                n222 = RT FIFO Delete(0:w196, 2:TRUE ("force destroy? (F)"), 3:w198) -> (11:w197:errorcluster)
                n223 = node-c288(w208) -> (w204:errorcluster)
                n224 = local read "Water duration (uS)"() -> (w155:u32)
                n225 = local read "Lick threshold (V)"() -> (w156:fxp<+,32,16>)
                n226 = RT FIFO Delete(0:w194, 2:TRUE ("force destroy? (F)"), 3:w193) -> (11:w192:errorcluster)
                n227 = node-c288("State machine cycle (uS)") -> (w211:T3)  [unwired: 3 in]
                n228 = local read "VS threshold (V)"() -> (w157:fxp<+,32,16>)
                n229 = local read "Water refractory period (uS)"() -> (w153:u32)
                n230 = local read "Shock refractory period (uS)"() -> (w154:u32)
                n231 = timed-loop {
                  timing: w211 -> [_]
                  timing-out: [_] -> w210
                  shift-right: [w433] -> _
                  shift-left: w152 -> [w444]
                  shift-right: [w434] -> _
                  shift-left: 1 -> [w445]
                  shift-right: [w432] -> _
                  shift-left: w152 -> [w439]
                  tunnel: w173 -> [w476]
                  shift-right: [w475] -> w200
                  shift-left: w172 -> [w474]
                  shift-right: [w435] -> _
                  shift-left: w195 -> [w446]
                  tunnel: w178 -> [w471]
                  shift-right: [w469] -> w191
                  shift-left: w177 -> [w470]
                  shift-right: [w472] -> _
                  shift-left: sgl[] [] ("array type (2D Dbl)") -> [w477]
                  tunnel: w144 -> [w462]
                  tunnel: [w455] -> w167
                  tunnel: w140 -> [w453]
                  tunnel: [w450] -> w165
                  tunnel: "VS filter period (uS)" -> [w417]
                  tunnel: w157 -> [w418]
                  tunnel: w156 -> [w448]
                  tunnel: w155 -> [w441]
                  tunnel: w154 -> [w436]
                  tunnel: w153 -> [w438]
                  shift-right: [w431] -> _
                  shift-left: w152 -> [w443]
                  tunnel: w151 -> [w416]
                  tunnel: w142 -> [w408]
                  tunnel: [w405] -> w145
                  shift-right: [w456] -> w168
                  shift-left: w143 -> [w461]
                  shift-right: [w406] -> w146
                  shift-left: w141 -> [w407]
                  shift-right: [w451] -> w164
                  shift-left: w139 -> [w452]
                  stop <- w463 stop-if-true
                  w429 = T1."Idle"
                  # "Ephys Trigger"
                  # "Pool 100 cycles"
                  # "ADD TRIAL #, Start and end of trial"
                  n232 = node-c288() -> (→"Actual cycle period (uS)":i64)  [unwired: 1 in, 1 out]
                  n233 = local read "Lick reward"() -> (w480:bool)
                  n234 = local read "Reward period (uS)"() -> (w442:u32)
                  n235 = call-poly <vilib>:"DAQmx Read.vi"("task/channels in"=w462, "timeout"=0.1, "error in"=w461) -> ("task out"=w455:refnum<k21>, "data"=w458:dbl[], "error out"=w456:errorcluster)  [unwired: 10 in]
                  n236 = call "Tick Count"() -> ("Tick Count(uSec)"=w488:u32)
                  n237 = Index Array(array=w458, index #1=0 ("index"), index #2=1 ("index"), index #3=2 ("index"), index #4=3 ("index"), index #5=4 ("index")) -> (element #1=w449:dbl, element #2=w457:dbl, element #3=w419:dbl, element #4=w415:dbl, element #5=w422:dbl)
                  n238 = feedback #1(FALSE) -> (w483:bool)
                  n239 = feedback-in #1(w480) -> ()
                  n240 = feedback #2(w488) -> (w489:u32)
                  n241 = feedback-in #2(w488) -> ()
                  n242 = local read "Trial timeout (uS)"() -> (w437:u32)
                  n243 = Greater?(x=w480, y=w483) -> (0:w481:bool)
                  n244 = local read "Pulse delay"() -> (w399:sgl)
                  n245 = Subtract(x=w488, y=w489) -> (x-y=w487:u32)
                  n246 = call "vs digital filter3.vi"("filter period(uSec)"=w417, "vs threshold"=w418, "input"=w419) -> ("output"=w414:bool)  [unwired: 3 in]
                  n247 = To Unsigned Quad Integer(1:w487) -> (0:w486:u64)
                  n248 = Greater?(x=w457, y=w448) -> (0:w413:bool)
                  n249 = feedback #3(u64 0) -> (w485:u64)
                  n250 = Add(x=w486, y=w485) -> (x+y=w440:u64)
                  n251 = Divide(x=w440, y=u64 1000) -> (x/y=w479:dbl)
                  n252 = feedback-in #3(w440) -> ()
                  n253 = call "vs digital filter.vi"("filter period(uSec)"=w417, "vs threshold"=w418, "input"=w449) -> ("output"=w396:bool)  [unwired: 3 in]
                  n254 = feedback #4(w429) -> (w490:T1)
                  n255 = Select(t=T1."Lick reward", s=w481, f=w490) -> (s? t:f=w425:T1)
                  n256 = feedback #5(w429) -> (w430:T1)
                  n257 = Multiply(x=w399, y=sgl 1000.0) -> (x*y=w398:sgl)
                  n258 = local read "ABORT"() -> (w463:bool)
                  n259 = local read "Pulse period (ms)"() -> (w402:sgl)
                  n260 = Build Array(w479, w445, w425, w415) -> (w411:dbl[])
                  n261 = To Single Precision Float(number=w411) -> (single precision float=w412:sgl[])
                  n262 = Multiply(x=w402, y=sgl 1000.0) -> (x*y=w401:sgl)
                  n263 = shared-variable "My Computer\\Network variables.lvlib\\stop - network"() -> (w491:bool)  [unwired: 1 in, 1 out]
                  n264 = call "vs digital filter2.vi"("filter period(uSec)"=w417, "vs threshold"=w418, "input"=w422) -> ("output"=w397:bool)  [unwired: 3 in]
                  n265 = case shown="\"VS\"" w425 {
                    selector: w425 -> [w505 w514 w529 w554 w564 w587 _ w609 w639 w666 _ w690 w698 w725]
                    tunnel: w446 -> [w506 w522 w537 w558 w581 w592 w603 w622 w643 w668 w683 w692 w710 w728]
                    tunnel: w445 -> [w502 w521 w536 w557 w579 w591 w602 w620 w642 w667 w682 w691 w709 w730]
                    tunnel: w413 -> [_ _ _ _ w567 _ _ _ _ _ _ _ _ w724]
                    tunnel: w444 -> [w501 w520 w535 w556 w571 w590 w599 w619 w629 w664 w680 w689 w704 w723]
                    tunnel: w443 -> [w500 w519 w533 w551 w577 w589 w598 w618 w635 w663 w679 w688 w707 w722]
                    tunnel: w442 -> [_ _ _ _ w575 _ _ _ _ _ _ _ _ _]
                    tunnel: w441 -> [_ _ _ _ _ _ _ w617 _ _ _ _ _ w721]
                    tunnel: w440 -> [_ _ _ w548 w570 _ _ w612 w632 w657 _ _ w701 w717]
                    tunnel: w439 -> [w499 w518 w534 w555 w576 w588 w597 w614 w634 w662 w670 w687 w706 w718]
                    tunnel: w398 -> [_ _ _ w549 _ _ _ _ _ _ _ _ _ _]
                    tunnel: w438 -> [_ _ _ _ _ _ _ _ _ _ _ _ _ _]
                    tunnel: w437 -> [_ _ _ _ _ _ _ _ w638 _ _ _ w702 _]
                    tunnel: w401 -> [_ _ _ _ _ _ _ _ _ w659 _ _ _ _]
                    tunnel: w436 -> [_ _ _ _ _ _ _ _ _ _ _ _ _ _]
                    tunnel: [w506 w522 w537 w558 w581 w592 w603 w621 w643 w668 w683 w692 w710 w729] -> w435
                    tunnel: [w502 w521 w536 w557 w579 w591 w601 w620 w642 w667 w682 w691 w709 w730] -> w434
                    tunnel: [w503 w517 w531 w541 w580 w587 T1."Idle" w611 w641 w650 w681 w690 w700 w726] -> w426
                    tunnel: [FALSE w511 w524 w538 w559 w584 w593 TRUE FALSE FALSE w669 w684 w693 w724] -> _
                    tunnel: [w501 w520 w535 w556 w569 w590 w599 w619 w629 w664 w680 w689 w697 w723] -> w433
                    tunnel: [w499 w518 w534 w555 w576 w588 w597 w613 w633 w654 w670 w687 w706 w715] -> w432
                    tunnel: [w500 w519 w533 w546 w577 w589 w598 w618 w635 w663 w679 w688 w707 w722] -> w431
                    tunnel: w430 -> [_ _ _ w553 w574 _ _ w624 w640 w665 _ _ w708 w727]
                    tunnel: w397 -> [_ w516 w530 w543 _ _ _ _ _ w653 w678 _ _ _]
                    tunnel: w408 -> [w496 w512 w525 w539 w560 w585 w594 w605 w626 w648 w676 w685 w695 w713]
                    tunnel: w407 -> [w497 w513 w526 w540 w561 w586 w595 w606 w627 w649 w675 w686 w694 w712]
                    tunnel: [w494 w512 w525 w539 w560 w585 w594 w605 w626 w647 w673 w685 w695 w713] -> w405
                    tunnel: [w493 w513 w526 w540 w561 w586 w595 w606 w627 w646 w672 w686 w694 w712] -> w406
                    tunnel: [FALSE w511 w524 w538 w559 w584 w593 FALSE FALSE TRUE w669 w684 w693 FALSE] -> w404
                    frame "Idle", Default {
                      n266 = local read "Start one trial"() -> (w504:bool)
                      n267 = call-poly <vilib>:"DAQmx Write.vi"("task/channels in"=w496, "data"=0.0, "error in"=w497) -> ("task out"=w494:refnum<k21>, "error out"=w493:errorcluster)  [unwired: 10 in, 1 out]
                      n268 = case shown="True" w504 {
                        tunnel: w505 -> [w507 _]
                        tunnel: [w507 w508] -> w503
                        frame False {
                        }
                        frame True {
                          n269 = stacked-sequence {
                            tunnel: [T1."Before VS" _] -> w508
                            frame #0 {
                            }
                            frame #1 {
                              w510 = FALSE
                              n270 = local write "Start one trial"(w510) -> ()
                              n271 = local write "Trial Done"(w510) -> ()
                            }
                          }
                        }
                      }
                    }
                    frame "Before VS" {
                      w511 = FALSE
                      n272 = Select(t=T1."VS", s=w516, f=w514) -> (s? t:f=w517:T1)
                    }
                    frame "VS" {
                      w524 = FALSE
                      n273 = local read "LED?"() -> (w523:bool)
                      n274 = Select(t=T1."VS2", s=w523, f=w529) -> (s? t:f=w528:T1)
                      n275 = Select(t=w528, s=w530, f=T1."Cycle End") -> (s? t:f=w531:T1)
                    }
                    frame "VS2" {
                      w538 = FALSE
                      # "Delay before LED!"
                      # "Punish=LED!!"
                      n276 = Equal?(x=w554, y=w553) -> (x = y?=w552:bool)
                      n277 = Add(x=w548, y=w549) -> (x+y=w550:sgl)
                      n278 = Select(t=w551, s=w552, f=w550) -> (s? t:f=w546:sgl)
                      n279 = Greater?(x=w546, y=w548) -> (0:w547:bool)
                      n280 = Select(t=w554, s=w547, f=T1."Punish") -> (s? t:f=w542:T1)
                      n281 = Select(t=w542, s=w543, f=T1."After VS") -> (s? t:f=w541:T1)
                    }
                    frame "After VS" {
                      w559 = FALSE
                      n282 = Equal?(x=w564, y=w574) -> (x = y?=w572:bool)
                      n283 = Add(x=w575, y=w570) -> (x+y=w573:u64)
                      n284 = Select(t=w571, s=w572, f=w573) -> (s? t:f=w569:u64)
                      n285 = Greater?(x=w569, y=w570) -> (0:w568:bool)
                      n286 = Select(t=T1."Reward", s=w567, f=w564) -> (s? t:f=w565:T1)
                      n287 = Select(t=w565, s=w568, f=T1."Cycle End") -> (s? t:f=w578:T1)
                      n288 = case shown="True" "Automatic reward" {
                        tunnel: [w582 T1."Reward"] -> w580
                        tunnel: w578 -> [w582 _]
                        frame False {
                        }
                        frame True {
                        }
                      }
                    }
                    frame "Wait for lever press" {
                      w584 = FALSE
                    }
                    frame "Cycle End" {
                      w593 = FALSE
                      n289 = Increment(x=w602) -> (x+1=w601:i32)
                      n290 = local write "Trial Done"(TRUE) -> ()
                    }
                    frame "Reward" {
                      n291 = Add(x=w617, y=w612) -> (x+y=w616:u64)
                      n292 = Increment(x=w622) -> (x+1=w623:i32)
                      n293 = Equal?(x=w609, y=w624) -> (x = y?=w615:bool)
                      n294 = Select(t=w614, s=w615, f=w616) -> (s? t:f=w613:sgl)
                      n295 = Select(t=w622, s=w615, f=w623) -> (s? t:f=w621:i32)
                      "# of rewards" <- w621
                      n296 = Greater?(x=w613, y=w612) -> (0:w610:bool)
                      n297 = Select(t=w609, s=w610, f=T1."Cycle End") -> (s? t:f=w611:T1)
                    }
                    frame "Reward Refractory" {
                      n298 = Equal?(x=w639, y=w640) -> (x = y?=w636:bool)
                      n299 = Add(x=w632, y=w638) -> (x+y=w637:u64)
                      n300 = Select(t=w634, s=w636, f=w637) -> (s? t:f=w633:sgl)
                      n301 = Greater?(x=w633, y=w632) -> (0:w631:bool)
                      n302 = Select(t=w639, s=w631, f=T1."Cycle End") -> (s? t:f=w641:T1)
                    }
                    frame "Punish" {
                      # "=LED!!"
                      n303 = Equal?(x=w666, y=w665) -> (x = y?=w661:bool)
                      n304 = local read "Pulse amp 0"() -> (w645:sgl)
                      n305 = Add(x=w657, y=w659) -> (x+y=w660:sgl)
                      n306 = Select(t=w662, s=w661, f=w660) -> (s? t:f=w654:sgl)
                      n307 = call-poly <vilib>:"DAQmx Write.vi"("task/channels in"=w648, "data"=w645, "error in"=w649) -> ("task out"=w647:refnum<k21>, "error out"=w646:errorcluster)  [unwired: 10 in, 1 out]
                      n308 = Greater?(x=w654, y=w657) -> (0:w658:bool)
                      n309 = Select(t=w666, s=w658, f=T1."Punish Refractory") -> (s? t:f=w651:T1)
                      n310 = Select(t=w651, s=w653, f=T1."Punish Refractory") -> (s? t:f=w650:T1)
                    }
                    frame "Punish Refractory" {
                      w669 = FALSE
                      # "Possibly code LED refractory period"
                      # "STOP LED HERE!"
                      n311 = call-poly <vilib>:"DAQmx Write.vi"("task/channels in"=w676, "data"=0.0, "error in"=w675) -> ("task out"=w673:refnum<k21>, "error out"=w672:errorcluster)  [unwired: 10 in, 1 out]
                      n312 = Select(t=T1."VS", s=w678, f=T1."After VS") -> (s? t:f=w681:T1)
                    }
                    frame "Exit" {
                      w684 = FALSE
                    }
                    frame "Timeout" {
                      w693 = FALSE
                      # "Can be used for pre-VS state for suppressing LED"
                      n313 = Equal?(x=w698, y=w708) -> (x = y?=w705:bool)
                      n314 = Add(x=w701, y=w702) -> (x+y=w703:u64)
                      n315 = Select(t=w704, s=w705, f=w703) -> (s? t:f=w697:u64)
                      n316 = Greater?(x=w697, y=w701) -> (0:w699:bool)
                      n317 = Select(t=w698, s=w699, f=T1."Cycle End") -> (s? t:f=w700:T1)
                    }
                    frame "Lick reward" {
                      n318 = Equal?(x=w725, y=w727) -> (x = y?=w720:bool)
                      n319 = Add(x=w721, y=w717) -> (x+y=w719:u64)
                      n320 = Select(t=w718, s=w720, f=w719) -> (s? t:f=w715:sgl)
                      n321 = Greater?(x=w715, y=w717) -> (0:w716:bool)
                      n322 = case shown="True" w724 {
                        tunnel: [w731 w733] -> w729
                        tunnel: w728 -> [w731 w732]
                        frame False {
                        }
                        frame True {
                          n323 = Increment(x=w732) -> (x+1=w733:i32)
                        }
                      }
                      n324 = Select(t=w725, s=w716, f=T1."Reward Refractory") -> (s? t:f=w726:T1)
                    }
                  }
                  n325 = Build Array(w414, w404, w396) -> (w466:bool[])
                  n326 = Boolean Array To Number(Boolean array=w466) -> (number=w409:u32)
                  n327 = To Single Precision Float(number=w409) -> (single precision float=w410:sgl)
                  n328 = Build Array (concatenate)(w412, w410) -> (w465:sgl[])
                  n329 = Build Array (concatenate)(w477, w465) -> (w473:sgl[])
                  n330 = Array Size(array=w473) -> (size(s)=w468:i32)
                  n331 = Equal?(x=w468, y=w416) -> (x = y?=w467:bool)
                  n332 = case shown="True" w467 {
                    tunnel: w476 -> [_ w746]
                    tunnel: [w736 w745] -> w475
                    tunnel: w474 -> [w736 w743]
                    tunnel: w473 -> [w735 w740]
                    tunnel: [w735 sgl[] [] ("array type (2D Dbl)")] -> w472
                    tunnel: w471 -> [_ w739]
                    tunnel: w470 -> [w734 w738]
                    tunnel: [w734 w737] -> w469
                    frame False {
                    }
                    frame True {
                      n333 = RT FIFO Write(0:w746, 1:w740, 2:10 ("timeout in ms (0)"), 3:w743) -> (11:w745:errorcluster)  [unwired: 1 in, 3 out]
                      n334 = RT FIFO Write(0:w739, 1:w740, 2:10 ("timeout in ms (0)"), 3:w738) -> (11:w737:errorcluster)  [unwired: 1 in, 3 out]
                    }
                  }
                  n335 = Select(t=T1."Exit", s=w491, f=w426) -> (s? t:f=w447:T1)
                  n336 = feedback-in #4(w447) -> ()
                  n337 = feedback-in #5(w447) -> ()
                  n338 = Build Array(w396, w397, w414) -> (w454:bool[])
                  n339 = node-c288() -> ()  [unwired: 3 in, 1 out]
                  n340 = call-poly <vilib>:"DAQmx Write.vi"("task/channels in"=w453, "data"=w454, "error in"=w452) -> ("task out"=w450:refnum<k21>, "error out"=w451:errorcluster)  [unwired: 10 in, 1 out]
                }
                n341 = node-c288(w210) -> (w203:errorcluster)
                n342 = call <vilib>:"DAQmx Stop Task.vi"("task/channels in"=w145, "error in"=w146) -> ("error out"=w147:errorcluster)  [unwired: 12 in, 1 out]
                n343 = call <vilib>:"DAQmx Stop Task.vi"("task/channels in"=w167, "error in"=w168) -> ("error out"=w166:errorcluster)  [unwired: 12 in, 1 out]
                n344 = Merge Errors(w197, w200, w192, w191) -> (w199:errorcluster)
                n345 = Build Array(w159, w159, w159) -> (w161:bool[])
                n346 = call-poly <vilib>:"DAQmx Write.vi"("task/channels in"=w165, "data"=w161, "error in"=w164) -> ("task out"=w163:refnum<k21>, "error out"=w162:errorcluster)  [unwired: 10 in, 1 out]
                n347 = call <vilib>:"DAQmx Stop Task.vi"("task/channels in"=w163, "error in"=w162) -> ("error out"=w181:errorcluster)  [unwired: 12 in, 1 out]
                n348 = Merge Errors(w166, w181, w147) -> (w201:errorcluster)
                n349 = stacked-sequence {
                  tunnel: w218 -> [w762]
                  tunnel: w219 -> [w761]
                  tunnel: w205 -> [w759]
                  tunnel: w204 -> [w758]
                  tunnel: w203 -> [w757]
                  tunnel: w201 -> [w756]
                  tunnel: w199 -> [w755]
                  frame #0 {
                    n350 = Merge Errors(w757, w758, w762, w761, w759, w756, w755) -> (w760:errorcluster)
                    "error out" <- w760
                    n351 = call <vilib>:"Simple Error Handler.vi"("error in (no error)"=w760) -> ()  [unwired: 4 in, 5 out]
                  }
                }
              }
            }
          }
          frame #2 {
            n352 = Wait (ms)(milliseconds to wait=u32 50) -> ()  [unwired: 1 out]
          }
        }
      }
      n353 = UDP Close(connection ID=w2, 8:w3) -> (error out=w1:errorcluster)  [unwired: 1 out]
      n354 = call <vilib>:"Simple Error Handler.vi"("error in (no error)"=w1) -> ()  [unwired: 4 in, 5 out]
    }
    frame #1 {
      w997 = FALSE
      n355 = local write "Busy"(w997) -> ()
      n356 = local write "ABORT"(w997) -> ()
      n357 = local write "Initial data received"(w997) -> ()
      n358 = local write "Stop state"(w997) -> ()
    }
  }
